vi "CCE RRMA P01 SubVI04.vi"(5 "ZB":i32, 7 "XB":i32, 8 "ZG":i32, 9 "XG":i32, 10 "ZR":i32, 11 "XR":i32) -> (3 "3D Picture":refnum<vi>(3d-picture))   [LabVIEW 2020]
doc: "Ceballos Conde Emanuel Rodríguez Ramírez Miguel Ángel 4MV6 Sistemas de visión artificial 2022/1\nEste vi genera una escena 3d en la cual se observan las camaras del sisitema de vision estereoscopica asi como el objeto u objetos detecados por dicho sistema"
uses:
  <vilib>/picture/3D Picture Control/Object/Create Object (drawable).vi
  <vilib>/picture/3D Picture Control/Object/Add Object (no reference).vi
  <vilib>/picture/3D Picture Control/NI_3D Picture Control.lvlib
panel:
  # "Ceballos Conde Emanuel\nRodríguez Ramírez Miguel Ángel\n4MV6\nSistemas de visión artificial\n2022/1"
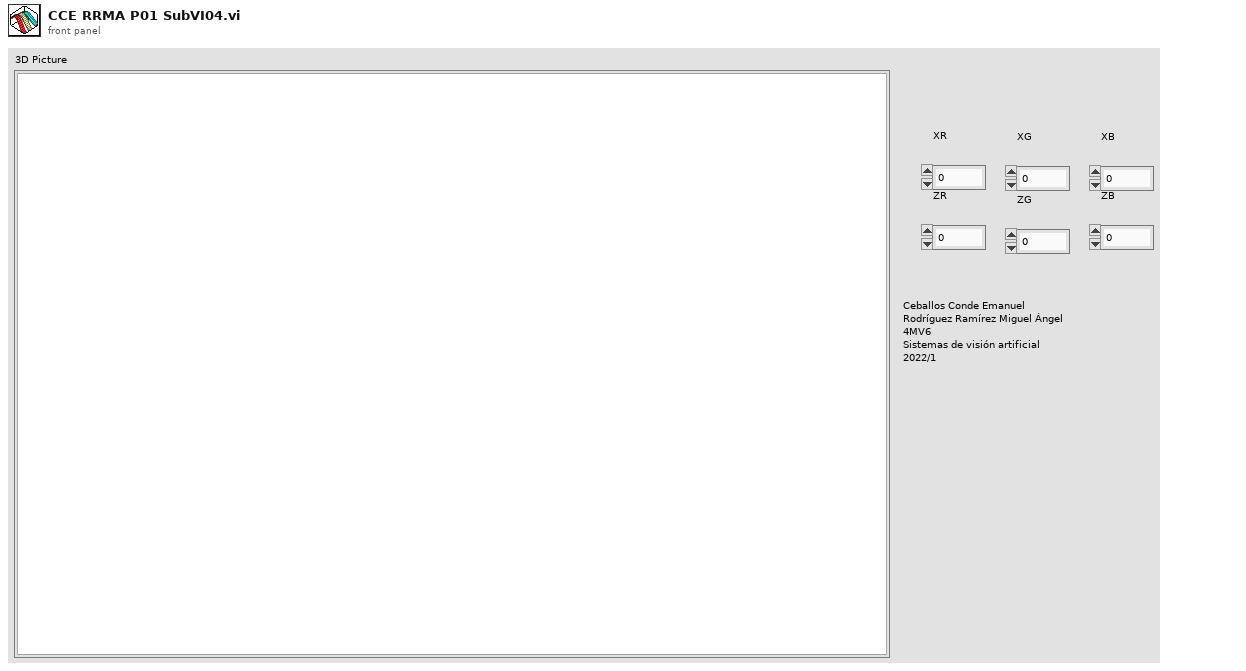
[diagram p1: front panel]
types:
  T1 = cluster{"Red":sgl, "Green":sgl, "Blue":sgl, "Alpha":sgl}
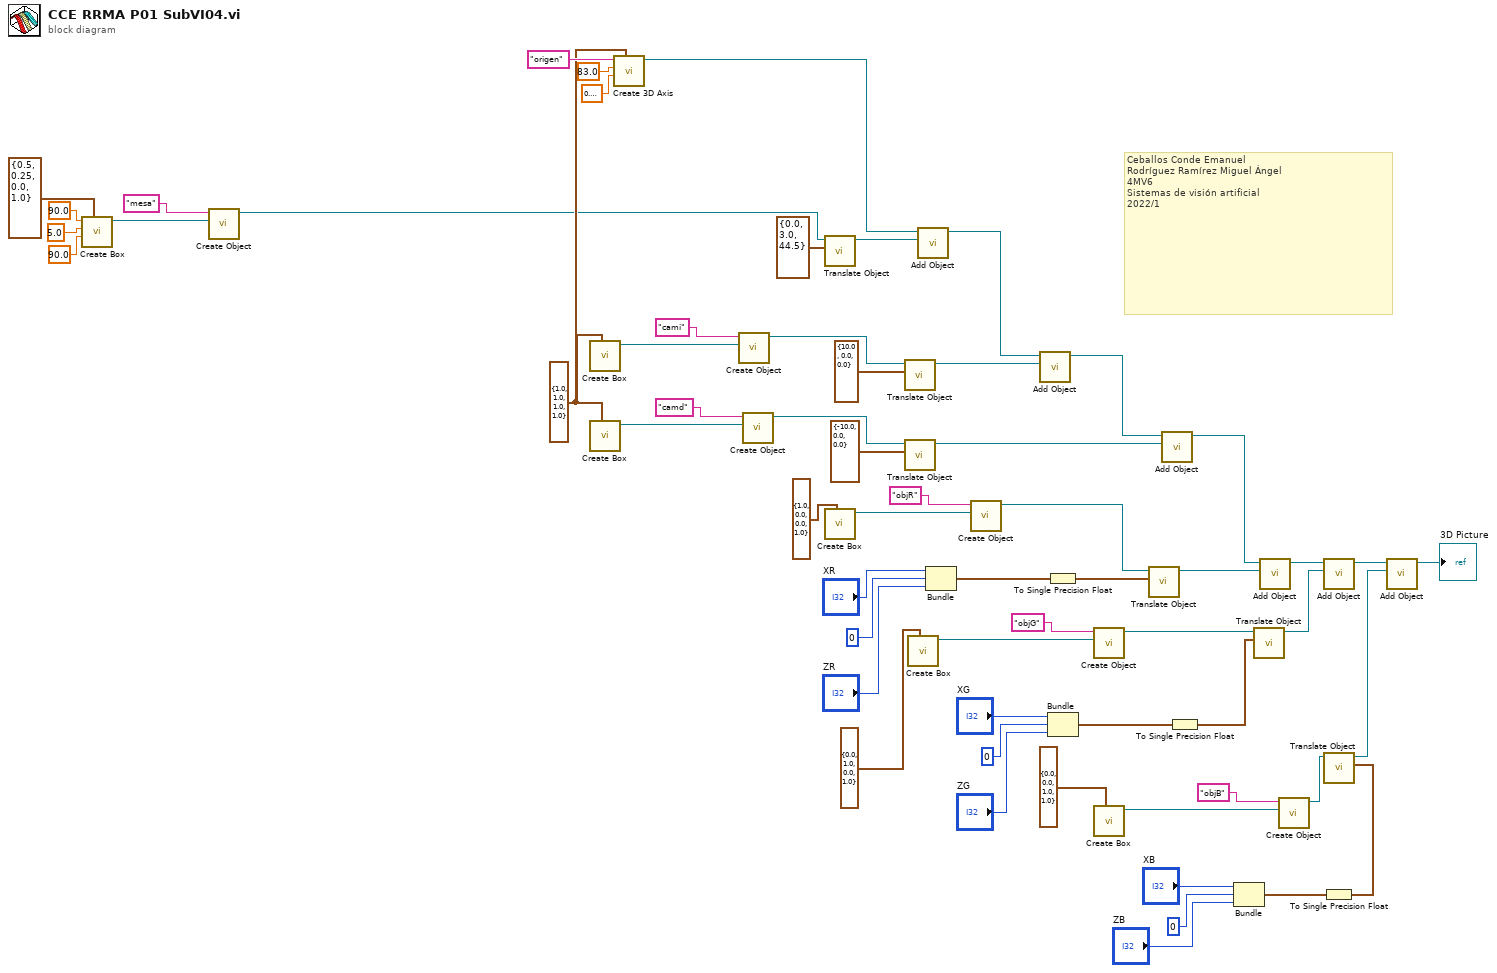
[diagram p0: block diagram]
diagram:
  w30 = T1 {"Red"=1.0, "Green"=1.0, "Blue"=1.0, "Alpha"=1.0} ("Color")
  # "Ceballos Conde Emanuel\nRodríguez Ramírez Miguel Ángel\n4MV6\nSistemas de visión artificial\n2022/1"
  n1 = call <vilib>:"Create Box.vi"("Color"=T1 {"Red"=0.5, "Green"=0.25, "Blue"=0.0, "Alpha"=1.0}, "Length Z"=sgl 90.0, "Length Y"=sgl 5.0, "Length X"=sgl 90.0) -> ("New Box Refnum"=w8:refnum<vi>)  [unwired: 6 in, 1 out]
  n2 = call-poly <vilib>:"Create Object.vi"("Geometry"=w8, "Name"="mesa") -> ("Scene:New Object"=w6:refnum<vi>)  [unwired: 8 in, 1 out]
  n3 = call <vilib>:"Create Box.vi"("Color"=w30) -> ("New Box Refnum"=w60:refnum<vi>)  [unwired: 9 in, 1 out]
  n4 = call <vilib>:"Create Box.vi"("Color"=w30) -> ("New Box Refnum"=w48:refnum<vi>)  [unwired: 9 in, 1 out]
  n5 = call <vilib>:"Create 3D Axis.vi"("Color"=w30, "Radius"=sgl 0.1, "Length"=sgl 83.0 ("Length X"), "Name"="origen") -> ("New Object Refnum"=w11:refnum<vi>)  [unwired: 6 in, 1 out]
  n6 = call-poly <vilib>:"Create Object.vi"("Geometry"=w60, "Name"="cami") -> ("Scene:New Object"=w58:refnum<vi>)  [unwired: 8 in, 1 out]
  n7 = call-poly <vilib>:"Create Object.vi"("Geometry"=w48, "Name"="camd") -> ("Scene:New Object"=w50:refnum<vi>)  [unwired: 8 in, 1 out]
  n8 = call <vilib>:"Translate Object.vi"("Translation"=cluster{"X":sgl, "Y":sgl, "Z":sgl} {"X"=0.0, "Y"=3.0, "Z"=44.5}, "Scene.Object In"=w6) -> ("Scene.Object Out"=w7:refnum<vi>)  [unwired: 8 in, 1 out]
  n9 = call <vilib>:"Create Box.vi"("Color"=T1 {"Red"=1.0, "Green"=0.0, "Blue"=0.0, "Alpha"=1.0}) -> ("New Box Refnum"=w46:refnum<vi>)  [unwired: 9 in, 1 out]
  n10 = call <vilib>:"Translate Object.vi"("Translation"=cluster{"X":sgl, "Y":sgl, "Z":sgl} {"X"=10.0, "Y"=0.0, "Z"=0.0}, "Scene.Object In"=w58) -> ("Scene.Object Out"=w57:refnum<vi>)  [unwired: 8 in, 1 out]
  n11 = call <vilib>:"Translate Object.vi"("Translation"=cluster{"X":sgl, "Y":sgl, "Z":sgl} {"X"=-10.0, "Y"=0.0, "Z"=0.0}, "Scene.Object In"=w50) -> ("Scene.Object Out"=w47:refnum<vi>)  [unwired: 8 in, 1 out]
  n12 = call <vilib>:"Create Box.vi"("Color"=T1 {"Red"=0.0, "Green"=1.0, "Blue"=0.0, "Alpha"=1.0}) -> ("New Box Refnum"=w36:refnum<vi>)  [unwired: 9 in, 1 out]
  n13 = call-poly <vilib>:"Add Object.vi"("New Object In"=w7, "Scene Object In"=w11) -> ("Scene Object Out"=w10:refnum<vi>)  [unwired: 8 in, 1 out]
  n14 = Bundle("XR"="XR", "element"=0, "ZR"="ZR") -> (w25:cluster{"XR":i32, "element":i32, "ZR":i32})  [unwired: 1 in]
  n15 = call-poly <vilib>:"Create Object.vi"("Geometry"=w46, "Name"="objR") -> ("Scene:New Object"=w44:refnum<vi>)  [unwired: 8 in, 1 out]
  n16 = call-poly <vilib>:"Add Object.vi"("New Object In"=w57, "Scene Object In"=w10) -> ("Scene Object Out"=w52:refnum<vi>)  [unwired: 8 in, 1 out]
  n17 = To Single Precision Float(number=w25) -> (single precision float=w14:cluster{"XR":sgl, "element":sgl, "ZR":sgl})
  n18 = Bundle("XG"="XG", "element"=0, "ZG"="ZG") -> (w19:cluster{"XG":i32, "element":i32, "ZG":i32})  [unwired: 1 in]
  n19 = call-poly <vilib>:"Create Object.vi"("Geometry"=w36, "Name"="objG") -> ("Scene:New Object"=w38:refnum<vi>)  [unwired: 8 in, 1 out]
  n20 = call <vilib>:"Create Box.vi"("Color"=T1 {"Red"=0.0, "Green"=0.0, "Blue"=1.0, "Alpha"=1.0}) -> ("New Box Refnum"=w35:refnum<vi>)  [unwired: 9 in, 1 out]
  n21 = call <vilib>:"Translate Object.vi"("Translation"=w14, "Scene.Object In"=w44) -> ("Scene.Object Out"=w39:refnum<vi>)  [unwired: 8 in, 1 out]
  n22 = call-poly <vilib>:"Add Object.vi"("New Object In"=w47, "Scene Object In"=w52) -> ("Scene Object Out"=w43:refnum<vi>)  [unwired: 8 in, 1 out]
  n23 = To Single Precision Float(number=w19) -> (single precision float=w13:cluster{"XG":sgl, "element":sgl, "ZG":sgl})
  n24 = Bundle("XB"="XB", "element"=0, "ZB"="ZB") -> (w15:cluster{"XB":i32, "element":i32, "ZB":i32})  [unwired: 1 in]
  n25 = call <vilib>:"Translate Object.vi"("Translation"=w13, "Scene.Object In"=w38) -> ("Scene.Object Out"=w32:refnum<vi>)  [unwired: 8 in, 1 out]
  n26 = call-poly <vilib>:"Add Object.vi"("New Object In"=w39, "Scene Object In"=w43) -> ("Scene Object Out"=w42:refnum<vi>)  [unwired: 8 in, 1 out]
  n27 = call-poly <vilib>:"Create Object.vi"("Geometry"=w35, "Name"="objB") -> ("Scene:New Object"=w33:refnum<vi>)  [unwired: 8 in, 1 out]
  n28 = call-poly <vilib>:"Add Object.vi"("New Object In"=w32, "Scene Object In"=w42) -> ("Scene Object Out"=w41:refnum<vi>)  [unwired: 8 in, 1 out]
  n29 = To Single Precision Float(number=w15) -> (single precision float=w12:cluster{"XB":sgl, "element":sgl, "ZB":sgl})
  n30 = call <vilib>:"Translate Object.vi"("Translation"=w12, "Scene.Object In"=w33) -> ("Scene.Object Out"=w31:refnum<vi>)  [unwired: 8 in, 1 out]
  n31 = call-poly <vilib>:"Add Object.vi"("New Object In"=w31, "Scene Object In"=w41) -> ("Scene Object Out"=→"3D Picture":refnum<vi>)  [unwired: 8 in, 1 out]
